vi "RQST Lookup Table.vi"(7 "Action":T2, 8 "error in (no error)":errorcluster, 10 "ID":u32, 11 "Data":T1) -> (0 "error out":errorcluster, 1 "Found?":bool, 3 "Data Out":T1)   [LabVIEW 2013, in "J1939.lvlib"]
uses:
  J1939.lvlib
  RQST Lookup Table Cluster.ctl
  <vilib>/xnet/xnet.llb/XNET Frame CAN.ctl
  <vilib>/xnet/xnet.llb/XNET Frame Type CAN.ctl
  RQST Lookup Table Action.ctl
panel:
  # "OUTPUTS"
  # "INPUTS"
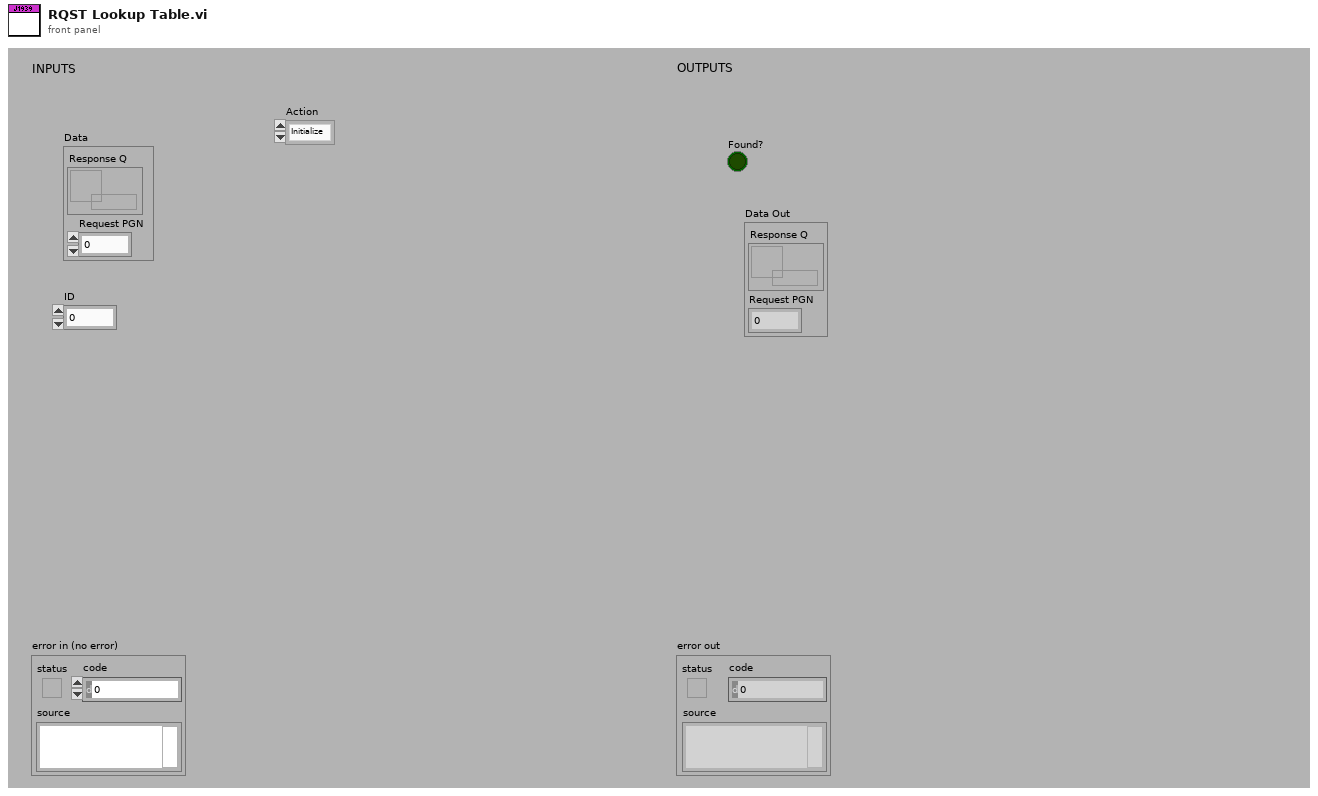
[diagram p1: front panel]
types:
  T1 = typedef "J1939.lvlib/RQST Lookup Table Cluster.ctl" = cluster{"Response Q":refnum<queue>, "Request PGN":u32}
  T2 = typedef "J1939.lvlib/RQST Lookup Table Action.ctl" = enum16{"Initialize", "Add", "Get", "Remove"}
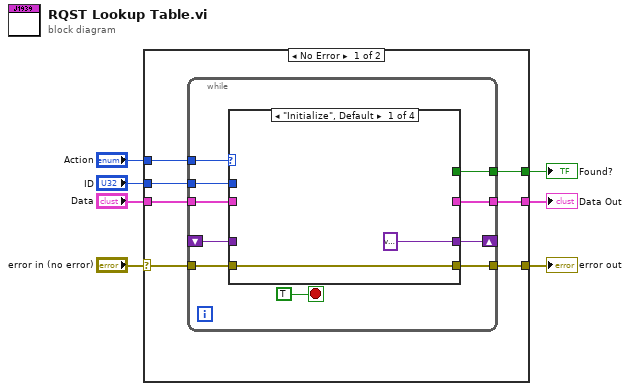
[diagram p0: block diagram]
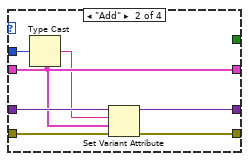
[diagram p2: hidden frame]
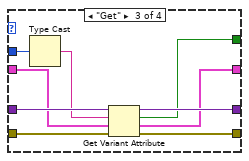
[diagram p3: hidden frame]
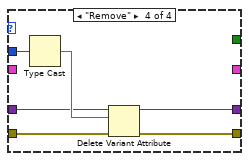
[diagram p4: hidden frame]
diagram:
  n1 = case shown="No Error" "error in (no error)" {
    selector: "error in (no error)" -> [w10 w49]
    tunnel: [w9 w49] -> w6
    tunnel: "Data" -> [w13 _]
    tunnel: "Action" -> [w14 _]
    tunnel: [w12 _] -> w3
    tunnel: "ID" -> [w11 _]
    tunnel: [w8 _] -> w1
    frame No Error {
      n2 = while {
        shift-right: [w23] -> _
        shift-left: _ -> [w21]
        tunnel: w14 -> [w24]
        tunnel: w13 -> [w22]
        tunnel: [w19] -> w12
        tunnel: w11 -> [w18]
        tunnel: w10 -> [w17]
        tunnel: [w16] -> w9
        tunnel: [w15] -> w8
        stop <- TRUE stop-if-true
        n3 = case shown="\"Initialize\", Default" w24 {
          tunnel: [variant ("duplicate variant") w32 w41 w43] -> w23
          tunnel: w22 -> [_ w31 w36 _]
          tunnel: w21 -> [_ w33 w42 w44]
          tunnel: [_ w31 w35 _] -> w19
          tunnel: w18 -> [_ w30 w40 w48]
          tunnel: w17 -> [w25 w28 w38 w47]
          tunnel: [w25 w27 w37 w46] -> w16
          tunnel: [_ _ w34 _] -> w15
          frame "Initialize", Default {
          }
          frame "Add" {
            n4 = Type Cast(x=w30) -> (*(type *) &x=w29:string)  [unwired: 1 in]
            n5 = Set Variant Attribute(Variant=w33, name=w29, value=w31, error in=w28) -> (Variant out=w32:variant, error out=w27:errorcluster)  [unwired: 1 out]
          }
          frame "Get" {
            n6 = Type Cast(x=w40) -> (*(type *) &x=w39:string)  [unwired: 1 in]
            n7 = Get Variant Attribute(Variant=w42, name=w39, default value (empty Variant)=w36, error in=w38) -> (duplicate Variant=w41:variant, found=w34:bool, value=w35:T1, error out=w37:errorcluster)
          }
          frame "Remove" {
            n8 = Type Cast(x=w48) -> (*(type *) &x=w45:string)  [unwired: 1 in]
            n9 = Delete Variant Attribute(4:w47, 6:w45, 7:w44) -> (0:w46:errorcluster, 3:w43:variant)  [unwired: 1 out]
          }
        }
      }
    }
    frame Error {
    }
  }
  "error out" <- w6
  "Data Out" <- w3
  "Found?" <- w1
